vi "Frame_acquisition.vi"(0 "Frames":T1=1, 5 "error in (no error)":errorcluster, 11 "Timeout":i32) -> (6 "FrameData":dbl[][][](array[numeric]), 10 "error out":errorcluster)   [LabVIEW 2020]
uses:
  Random subVIs/Control 1.ctl
panel:
  out "ExtChData":dbl[][](array[numeric])
  in  "ExChs":i32
  in  "Acq Trigger?":bool=TRUE
  # "IMAGE SETTINGS"
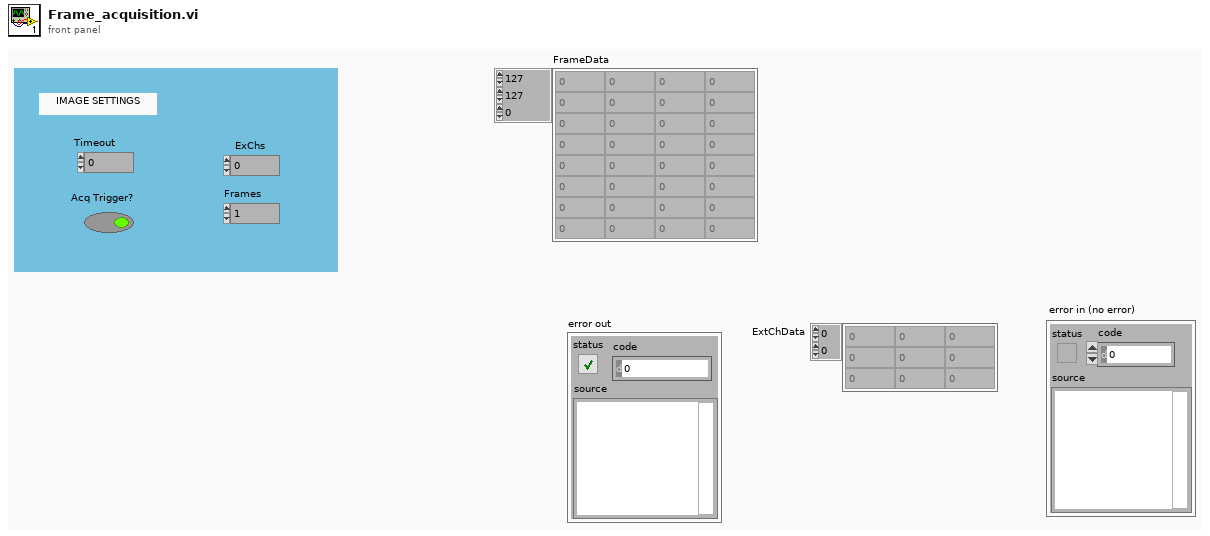
[diagram p1: front panel]
types:
  T1 = typedef "Control 1.ctl" = i32
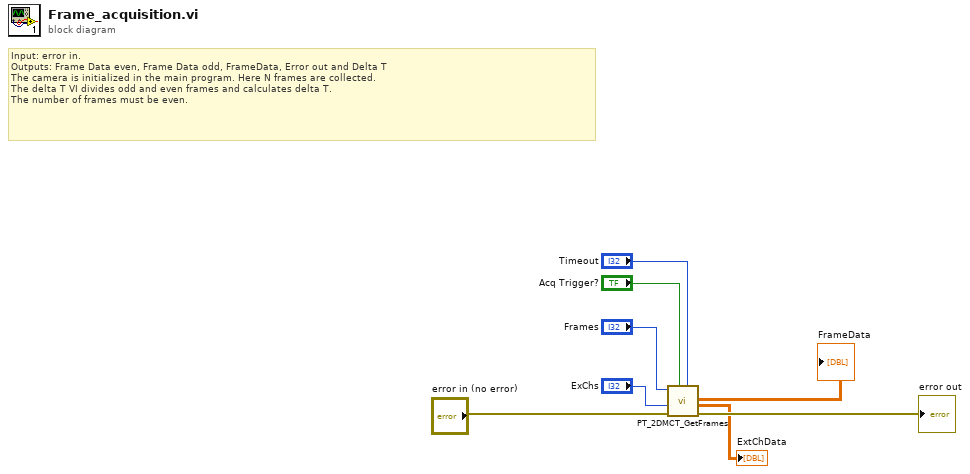
[diagram p0: block diagram]
diagram:
  # "Input: error in.\nOutputs: Frame Data even, Frame Data odd, FrameData, Error out and Delta T\nThe camera is initialized in the main program. Here N frames are collected.\nThe delta T VI divides odd and even frames and calculates delta T.\nThe number of frames must be even."
  n1 = call "PT_2DMCT_GetFrames.vi"("Timeout"="Timeout", "Acq Trigger?"="Acq Trigger?", "error in (no error)"="error in (no error)", "ExChs"="ExChs", "Frames"="Frames") -> ("error out"=→"error out":errorcluster, "ExtChData"=→"ExtChData":dbl[][], "FrameData"=→"FrameData":dbl[][][])  [unwired: 4 in]
